vi "Loop_ACT.vi"() -> ()   [LabVIEW 2017, in "Drive.lvlib"]
uses:
  Drive.lvlib
  <vilib>/Rock Robotics/WPI/MotorControl/WPI_MotorControlDeviceRef.ctl
  <vilib>/Rock Robotics/WPI/MotorControl/WPI_MotorControlType.ctl
  <vilib>/Rock Robotics/SystemInterfaces/DIO/FPGA_DIOPWMChannel.ctl
  <vilib>/Rock Robotics/WPI/PWM/WPI_PWMDeadband.ctl
  <vilib>/Rock Robotics/SystemInterfaces/DIO/FPGA_DIOChannel.ctl
  _SOURCE2018_Master/_SHARE ALL/RoboRio Share All/SRX Share All/TypeDefs SRX/Cluster_SRX_Mode and Value.ctl
  _SOURCE2018_Master/System Drivers/Phoenix-LabVIEW/Motor Controller/Controls/CTRE_Phoenix_MotorControl_ControlMode.ctl
  _SOURCE2018_Master/_SHARE ALL/RoboRio Share All/SRX Share All/TypeDefs SRX/Cluster_SRX_Config Voltage Output.ctl
  _SOURCE2018_Master/System Drivers/Phoenix-LabVIEW/Motor Controller/Controls/CTRE_Phoenix_MotorControl_NeutralMode.ctl
  _SOURCE2018_Master/_SHARE ALL/RoboRio Share All/SRX Share All/TypeDefs SRX/Cluster_SRX_Forward and Reverse.ctl
  _SOURCE2018_Master/_SHARE ALL/Global Share All/Global_STOP.vi
  Globals/CMD_Global.vi
panel:
  out "Output Data":dbl
  out "Input Data":dbl
  out "Cycle Time (S)":dbl format="%.3g"
  in  "Target Time(ms)":u32=50
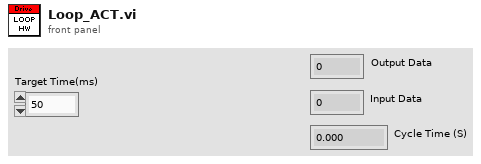
[diagram p1: front panel]
types:
  T1 = typedef "Cluster_SRX_Config Voltage Output.ctl" = cluster{"Invert?":bool, "Neutral Mode":T2, "Deadband (-1to1)":dbl, "Ramp Time Off to Full (S)":dbl, "Max Voltage (-1to1)":T3, "Min Voltage (-1to1":T3}
  T2 = typedef "CTRE_Phoenix_MotorControl_NeutralMode.ctl" = enum8{"EEPROMSetting", "Override to Coast", "Override to Brake"}
  T3 = typedef "Cluster_SRX_Forward and Reverse.ctl" = cluster{"Forward":dbl, "Reverse":dbl}
  T4 = typedef "Cluster_SRX_Mode and Value.ctl" = cluster{"Mode":T5, "Value":dbl}
  T5 = typedef "CTRE_Phoenix_MotorControl_ControlMode.ctl" = u16
  T6 = typedef "WPI_MotorControlDeviceRef.ctl" = cluster{"DeviceStatus":errorcluster, "Type":T7, "PWM":cluster{"PWM Channel":T8, "DeadBand":T9}, "CAN":cluster{"Device Number":u8, "SetOutput VI Ref":variant, "GetOutput VI Ref":variant, "Enable VI Ref":variant, "Disable VI Ref":variant, "Data":variant}, "Invert":bool, "DIO PWM":cluster{"PWM \"Enable\" Channel":T8, "DIOChannel":T10, "PWM Rate":dbl}}
  T7 = typedef "WPI_MotorControlType.ctl" = enum16{"PWM", "CAN", "DIO PWM"}
  T8 = typedef "FPGA_DIOPWMChannel.ctl" = enum8{"PWM 0", "PWM 1", "PWM 2", "PWM 3", "PWM 4", "PWM 5", "PWM 6", "PWM 7", "PWM 8", "PWM 9", "PWM MXP 0", "PWM MXP 1", "PWM MXP 2", "PWM MXP 3", "PWM MXP 4", "PWM MXP 5", "PWM MXP 6", "PWM MXP 7", "PWM MXP 8", "PWM MXP 9", "Invalid"}
  T9 = typedef "WPI_PWMDeadband.ctl" = cluster{"Name":string, "maxPositivePwm":i32, "minPositivePwm":i32, "centerPwm":i32, "maxNegativePwm":i32, "minNegativePwm":i32, "angularRange":u16}
  T10 = typedef "FPGA_DIOChannel.ctl" = enum8{"DIO 0", "DIO 1", "DIO 2", "DIO 3", "DIO 4", "DIO 5", "DIO 6", "DIO 7", "DIO 8", "DIO 9", "DIO MXP 0", "DIO MXP 1", "DIO MXP 2", "DIO MXP 3", "DIO MXP 4", "DIO MXP 5", "DIO MXP 6", "DIO MXP 7", "DIO MXP 8", "DIO MXP 9", "DIO MXP 10", "DIO MXP 11", "DIO MXP 12", "DIO MXP 13", "DIO MXP 14", "DIO MXP 15", "SPI Port CS1", "SPI Port CS2", "SPI Port CS3", "SPI Port MISO", "SPI Port MOSI", "Invalid"}
  T11 = cluster{"Left Motor Ref":T6, "Right Motor Ref":T6, " Motor Values":dbl, "Actuator Input":dbl, "Target Time(ms)":u32, "Current Time":timestamp, "Previous Time":timestamp, "Cycle Time (S)":dbl, "CMD_LeftMotor ":T4, "CMD_RightMotor":T4}
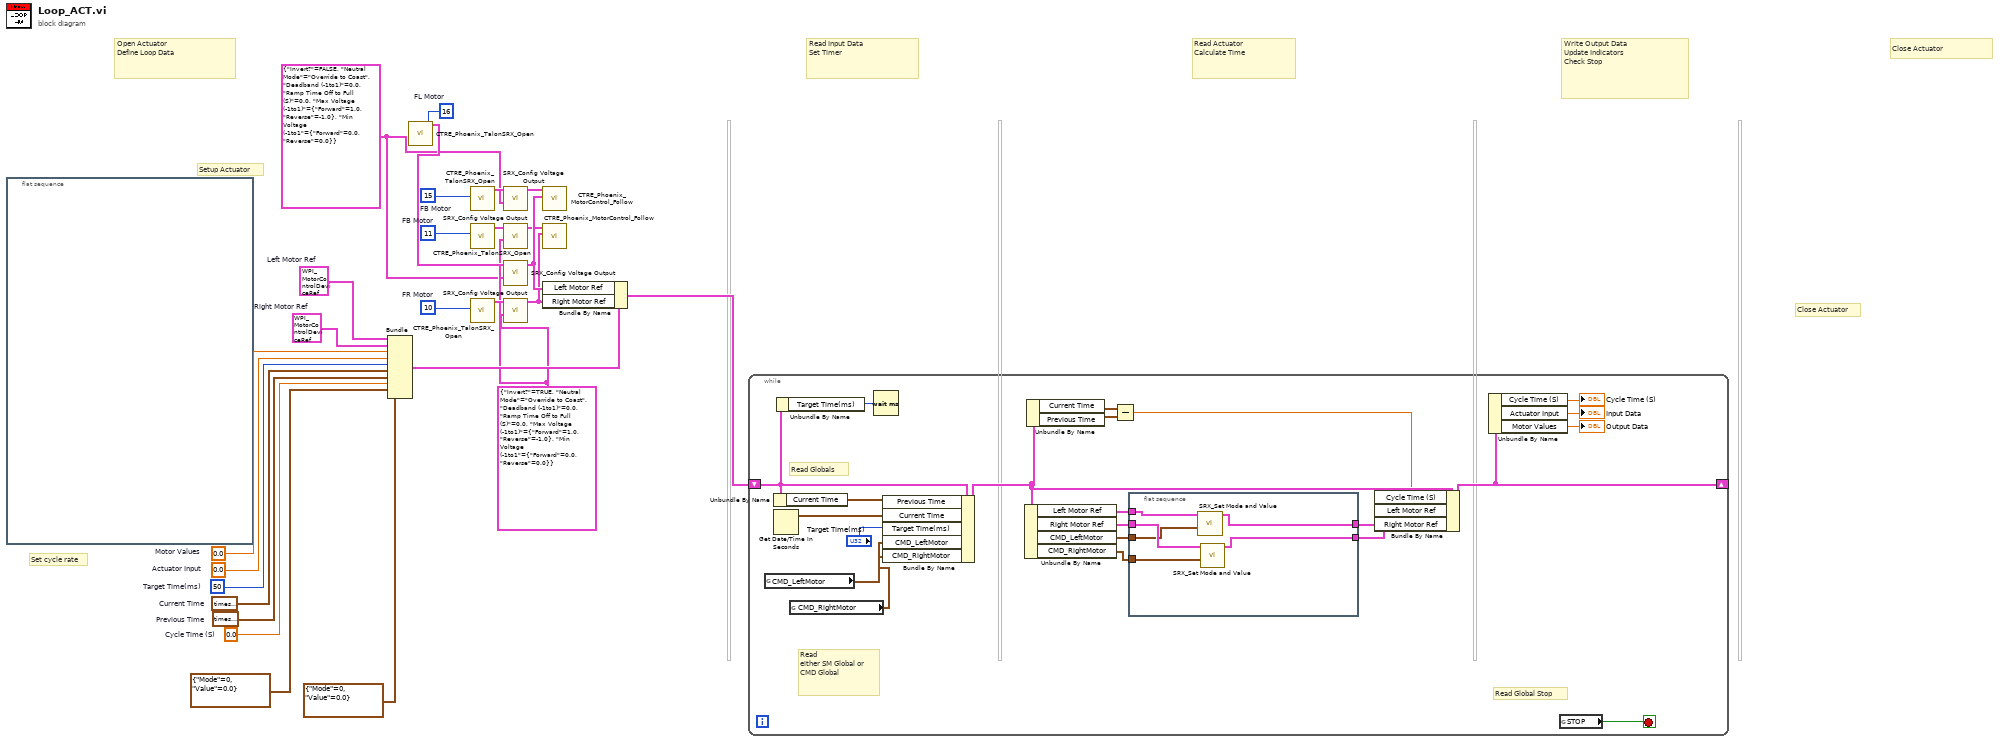
[diagram p0: block diagram]
diagram:
  w10 = u8 11  # FB Motor
  w11 = u8 15  # FB Motor
  w4 = T1 {"Invert?"=TRUE, "Neutral Mode"=enum."Override to Coast", "Deadband (-1to1)"=0.0, "Ramp Time Off to Full (S)"=0.0, "Max Voltage (-1to1)"={"Forward"=1.0, "Reverse"=-1.0}, "Min Voltage (-1to1"={"Forward"=0.0, "Reverse"=0.0}} ("Output Config")
  w1 = T1 {"Invert?"=FALSE, "Neutral Mode"=enum."Override to Coast", "Deadband (-1to1)"=0.0, "Ramp Time Off to Full (S)"=0.0, "Max Voltage (-1to1)"={"Forward"=1.0, "Reverse"=-1.0}, "Min Voltage (-1to1"={"Forward"=0.0, "Reverse"=0.0}} ("Output Config")
  w15 = u8 10  # FR Motor
  w16 = u8 16  # FL Motor
  w20 = T6 {"DeviceStatus"={"status"=FALSE, "code"=0, "source"=""}, "Type"=enum."PWM", "PWM"={"PWM Channel"=enum."PWM 1", "DeadBand"={"Name"="", "maxPositivePwm"=0, "minPositivePwm"=0, "centerPwm"=0, "maxNegativePwm"=0, "minNegativePwm"=0, "angularRange"=0}}, "CAN"={"Device Number"=0, "SetOutput VI Ref"=variant(enum8{"Percent VBus", "Current", "Speed", "Position", "Voltage"} enum."Percent VBus"), "GetOutput VI Ref"=variant(refnum<k1> refnum), "Enable VI Ref"=variant(dbl 12.0), "Disable VI Ref"=variant(enum8{"Percent VBus", "Speed", "Position", "Slave", "Unchanged / Invalid", "Voltage Compensation", "Current", "Motion Profile"} enum."Percent VBus"), "Data"=variant}, "Invert"=FALSE, "DIO PWM"={"PWM \"Enable\" Channel"=enum."Invalid", "DIOChannel"=enum."Invalid", "PWM Rate"=0.0}}  # Right Motor Ref
  w19 = T6 {"DeviceStatus"={"status"=FALSE, "code"=0, "source"=""}, "Type"=enum."PWM", "PWM"={"PWM Channel"=enum."PWM 1", "DeadBand"={"Name"="", "maxPositivePwm"=0, "minPositivePwm"=0, "centerPwm"=0, "maxNegativePwm"=0, "minNegativePwm"=0, "angularRange"=0}}, "CAN"={"Device Number"=0, "SetOutput VI Ref"=variant(enum8{"Percent VBus", "Current", "Speed", "Position", "Voltage"} enum."Percent VBus"), "GetOutput VI Ref"=variant(refnum<k1> refnum), "Enable VI Ref"=variant(dbl 12.0), "Disable VI Ref"=variant(enum8{"Percent VBus", "Speed", "Position", "Slave", "Unchanged / Invalid", "Voltage Compensation", "Current", "Motion Profile"} enum."Percent VBus"), "Data"=variant}, "Invert"=FALSE, "DIO PWM"={"PWM \"Enable\" Channel"=enum."Invalid", "DIOChannel"=enum."Invalid", "PWM Rate"=0.0}}  # Left Motor Ref
  w21 = 0.0  # Cycle Time (S)
  w26 = timestamp(0 s since 1904-01-01)  # Previous Time
  w25 = timestamp(0 s since 1904-01-01)  # Current Time
  w24 = u32 50  # Target Time(ms)
  w23 = 0.0  # Actuator Input
  w22 = 0.0  # Motor Values
  # "Close Actuator"
  # "Write Output Data\nUpdate Indicators\nCheck Stop"
  # "Read Actuator\nCalculate Time"
  # "Read Input Data\nSet Timer"
  # "Open Actuator\nDefine Loop Data"
  # "Set cycle rate"
  # "Close Actuator"
  # "Setup Actuator"
  n1 = flat-sequence {
    frame #0 {
    }
  }
  n2 = Bundle("Left Motor Ref"=w19, "Right Motor Ref"=w20, "Motor Values"=w22, "Actuator Input"=w23, "Target Time(ms)"=w24, "Current Time"=w25, "Previous Time"=w26, "Cycle Time (S)"=w21, "CMD_LeftMotor"=T4 {"Mode"=0, "Value"=0.0}, "CMD_RightMotor"=T4 {"Mode"=0, "Value"=0.0}) -> (w18:T11)  [unwired: 1 in]
  n3 = call "CTRE_Phoenix_TalonSRX_Open.vi"("Device Number"=w16) -> ("CAN Talon SRX Ref"=w12:T6)  [unwired: 9 in, 1 out]
  n4 = call "CTRE_Phoenix_TalonSRX_Open.vi"("Device Number"=w11) -> ("CAN Talon SRX Ref"=w3:T6)  [unwired: 9 in, 1 out]
  n5 = call "CTRE_Phoenix_TalonSRX_Open.vi"("Device Number"=w10) -> ("CAN Talon SRX Ref"=w6:T6)  [unwired: 9 in, 1 out]
  n6 = call "CTRE_Phoenix_TalonSRX_Open.vi"("Device Number"=w15) -> ("CAN Talon SRX Ref"=w9:T6)  [unwired: 9 in, 1 out]
  n7 = call "SRX_Config Voltage Output.vi"("Output Config"=w1, "PhoenixMotorControlDevRef"=w3) -> ("PhoenixMotorControlDevRef Out"=w2:T6)  [unwired: 8 in, 1 out]
  n8 = call "SRX_Config Voltage Output.vi"("Output Config"=w4, "PhoenixMotorControlDevRef"=w6) -> ("PhoenixMotorControlDevRef Out"=w5:T6)  [unwired: 8 in, 1 out]
  n9 = call "SRX_Config Voltage Output.vi"("Output Config"=w1, "PhoenixMotorControlDevRef"=w12) -> ("PhoenixMotorControlDevRef Out"=w8:T6)  [unwired: 8 in, 1 out]
  n10 = call "SRX_Config Voltage Output.vi"("Output Config"=w4, "PhoenixMotorControlDevRef"=w9) -> ("PhoenixMotorControlDevRef Out"=w7:T6)  [unwired: 8 in, 1 out]
  n11 = call "CTRE_Phoenix_MotorControl_Follow.vi"("Master Controller to Follow"=w8, "PhoenixMotorControlDevRef"=w2) -> ()  [unwired: 8 in, 2 out]
  n12 = call "CTRE_Phoenix_MotorControl_Follow.vi"("Master Controller to Follow"=w7, "PhoenixMotorControlDevRef"=w5) -> ()  [unwired: 8 in, 2 out]
  n13 = Bundle By Name(cluster=w18, "Left Motor Ref"=w8, "Right Motor Ref"=w7) -> (w17:T11)
  n14 = while {
    shift-right: [w38] -> _
    shift-left: w17 -> [w40]
    stop <- w48 stop-if-true
    # "Read\neither SM Global or CMD Global"
    # "Read Globals"
    # "Read Global Stop"
    n15 = global read "CMD_Global.vi" "CMD_LeftMotor"() -> (w30:T4)
    n16 = Unbundle By Name(w40) -> ("Current Time"=w45:timestamp)
    n17 = Get Date/Time In Seconds() -> (seconds since 1Jan1904=w46:timestamp)
    n18 = Unbundle By Name(w40) -> ("Target Time(ms)"=w39:u32)
    n19 = global read "CMD_Global.vi" "CMD_RightMotor"() -> (w29:T4)
    n20 = Wait (ms)(milliseconds to wait=w39) -> ()  [unwired: 1 out]
    n21 = Bundle By Name(cluster=w40, "Previous Time"=w45, "Current Time"=w46, "Target Time(ms)"="Target Time(ms)", "CMD_LeftMotor"=w30, "CMD_RightMotor"=w29) -> (w41:T11)
    n22 = Unbundle By Name(w41) -> ("Left Motor Ref"=w47:T6, "Right Motor Ref"=w33:T6, "CMD_LeftMotor"=w28:T4, "CMD_RightMotor"=w27:T4)
    n23 = Unbundle By Name(w41) -> ("Current Time"=w44:timestamp, "Previous Time"=w43:timestamp)
    n24 = Subtract(x=w44, y=w43) -> (x-y=w34:dbl)
    n25 = flat-sequence {
      tunnel: w47 -> [w54]
      tunnel: w33 -> [w53]
      tunnel: [w52] -> w32
      tunnel: [w51] -> w31
      tunnel: w28 -> [w50]
      tunnel: w27 -> [w49]
      frame #0 {
        n26 = call "SRX_Set Mode and Value.vi"("Mode And Value"=w50, "PhoenixMotorControlDevRef"=w54) -> ("PhoenixMotorControlDevRef Out"=w51:T6)  [unwired: 8 in, 1 out]
        n27 = call "SRX_Set Mode and Value.vi"("Mode And Value"=w49, "PhoenixMotorControlDevRef"=w53) -> ("PhoenixMotorControlDevRef Out"=w52:T6)  [unwired: 8 in, 1 out]
      }
    }
    n28 = Bundle By Name(cluster=w41, "Cycle Time (S)"=w34, "Left Motor Ref"=w31, "Right Motor Ref"=w32) -> (w38:T11)
    n29 = Unbundle By Name(w38) -> ("Cycle Time (S)"=→"Cycle Time (S)":dbl, "Actuator Input"=→"Input Data":dbl, "Motor Values"=→"Output Data":dbl)
    n30 = global read "Global_STOP.vi" "STOP"() -> (w48:bool)
  }
